vi "Initialize FPGA Starter Kit Host.vi"(7 "run FPGA (T)":bool=TRUE, 8 "error in (no error)":errorcluster, 10 "IP address (\"\")":string, 11 "FPGA starter kit host in":refnum<class "NI_Robotics_Starter Kit Host_FPGA.lvclass">) -> (0 "error out":errorcluster, 3 "FPGA starter kit host out":refnum<class "NI_Robotics_Starter Kit Host_FPGA.lvclass">)   [LabVIEW 2017, in "NI_Robotics_Starter Kit Host_FPGA.lvclass"]
uses:
  <vilib>/robotics/Starter Kit/FPGA Host Interface/NI_Robotics_Starter Kit Host_FPGA.lvclass
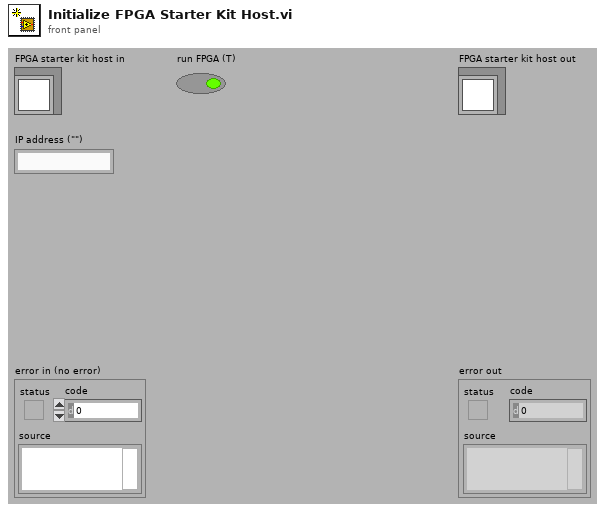
[diagram p1: front panel]
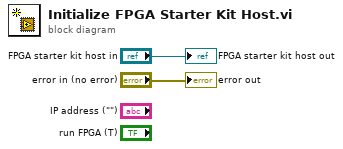
[diagram p0: block diagram]
diagram:
  "error out" <- "error in (no error)"
  "FPGA starter kit host out" <- "FPGA starter kit host in"
